vi "Billard2020.vi"() -> ()   [LabVIEW 2019]
uses:
  <vilib>/picture/picture.llb/imagedata.ctl
panel:
  in  "line":string
  in  "ball touch":u32(colorbox)
  in  "band touch":u32(colorbox)
  in  "Script":string
  out "ML":string
  out "return code":i32
  in  "Blue BG":T1={"Rmin"=39, "Rmax"=62, "Gmin"=91, "Gmax"=116, "Bmin"=202, "Bmax"=255}
  in  "White Ball":T1={"Rmin"=100, "Rmax"=255, "Gmin"=100, "Gmax"=255, "Bmin"=100, "Bmax"=255}
  in  "Yellow Ball":T1={"Rmin"=140, "Rmax"=255, "Gmin"=140, "Gmax"=255, "Bmin"=0, "Bmax"=175}
  in  "Red Ball":T1={"Rmin"=160, "Rmax"=255, "Gmin"=0, "Gmax"=160, "Bmin"=0, "Bmax"=160}
  in  "Dark Blue frame":T2={"Rmin"=0, "Gmin"=0, "Bmin"=121, "Rmax"=14, "Gmax"=42, "Bmax"=126}
  out "Bords du billard":T3
  out "filenames":string[](array[string])
  in  "path":path
  out "error out":errorcluster
  out "Ball coordinates":string
  out "standard error":string
  out "standard output":string
  out "appended array":u32[](array[numeric])
  out "H":i16
  out "W":i16
  out "2D Picture":picture
  out "image data":T4
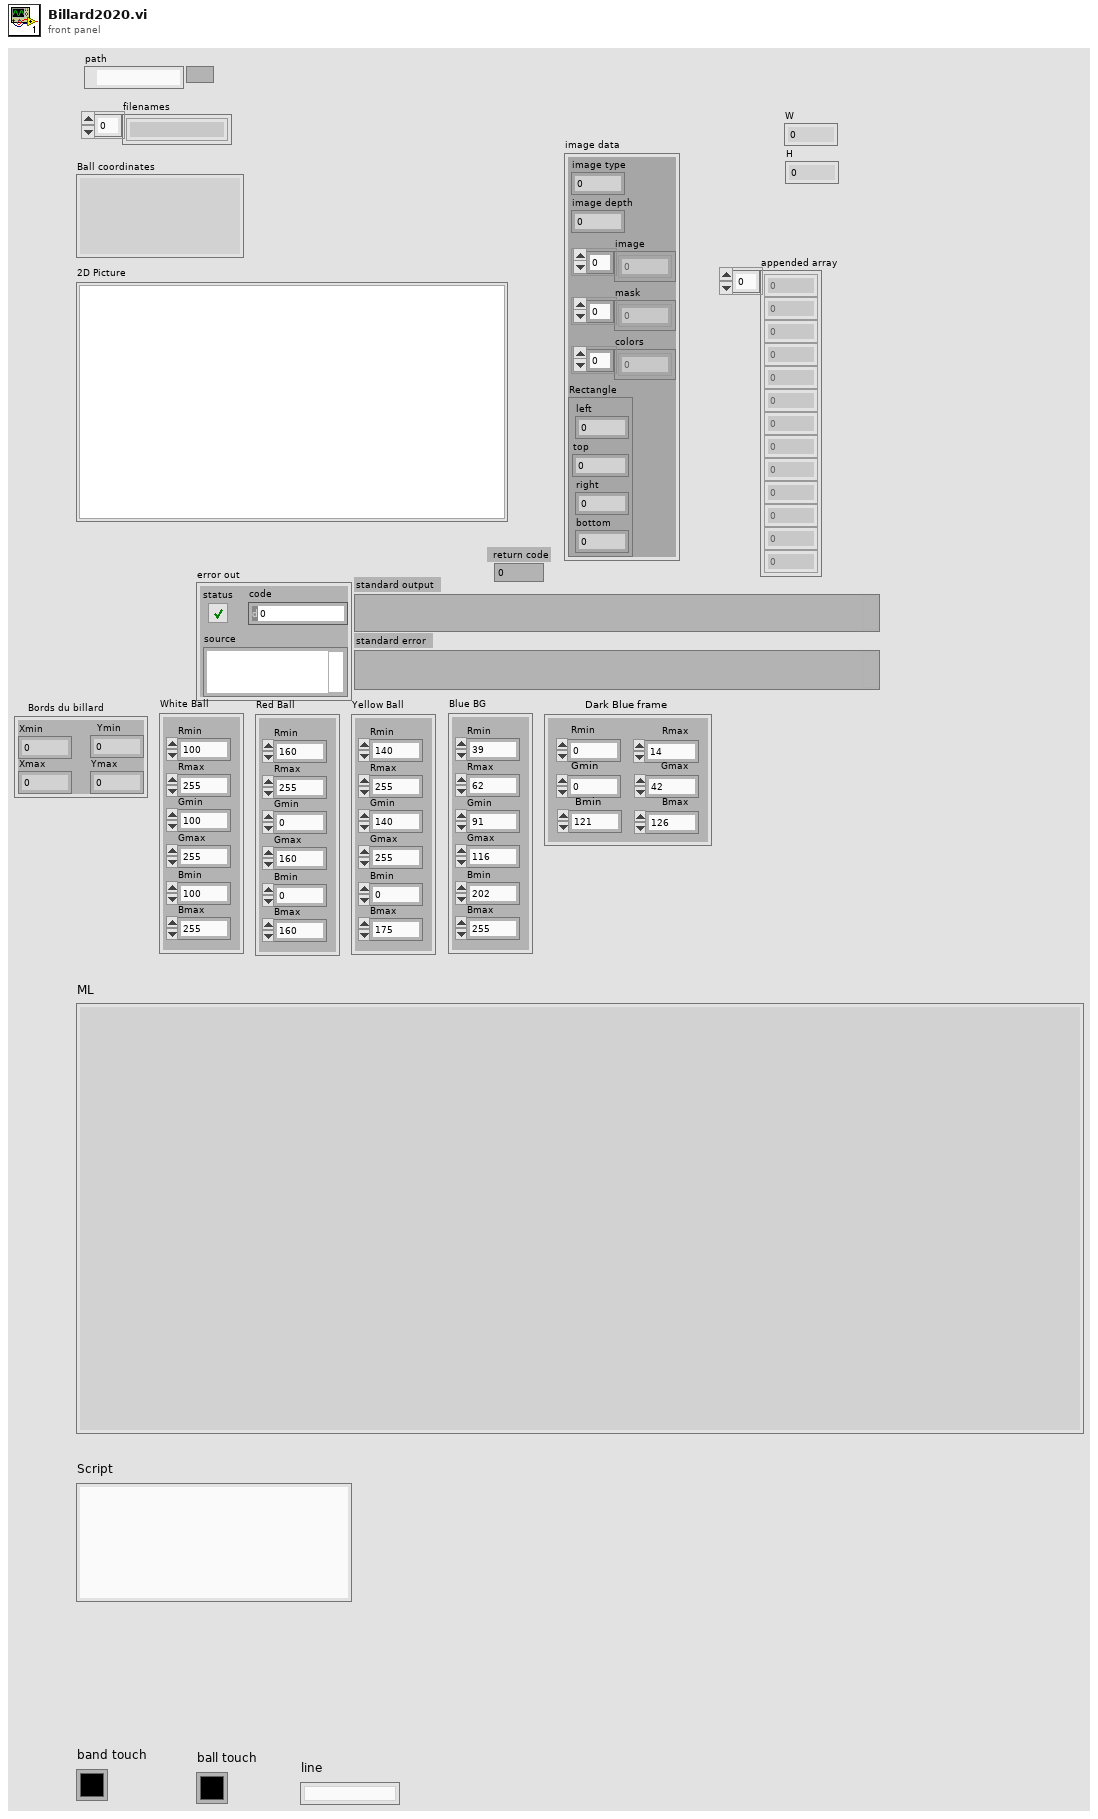
[diagram p1: front panel]
types:
  T1 = cluster{"Rmin":i32, "Rmax":i32, "Gmin":i32, "Gmax":i32, "Bmin":i32, "Bmax":i32}
  T2 = cluster{"Rmin":u32, "Gmin":u32, "Bmin":u32, "Rmax":u32, "Gmax":u32, "Bmax":u32}
  T3 = cluster{"Xmin":i32, "Ymin":i32, "Xmax":i32, "Ymax":i32}
  T4 = typedef "imagedata.ctl" = cluster{"image type":i32, "image depth":i32, "image":u8[], "mask":u8[], "colors":u32[], "Rectangle":cluster{"left":i16, "top":i16, "right":i16, "bottom":i16}}
  T5 = enum16{"big-endian, network order", "native, host order", "little-endian"}
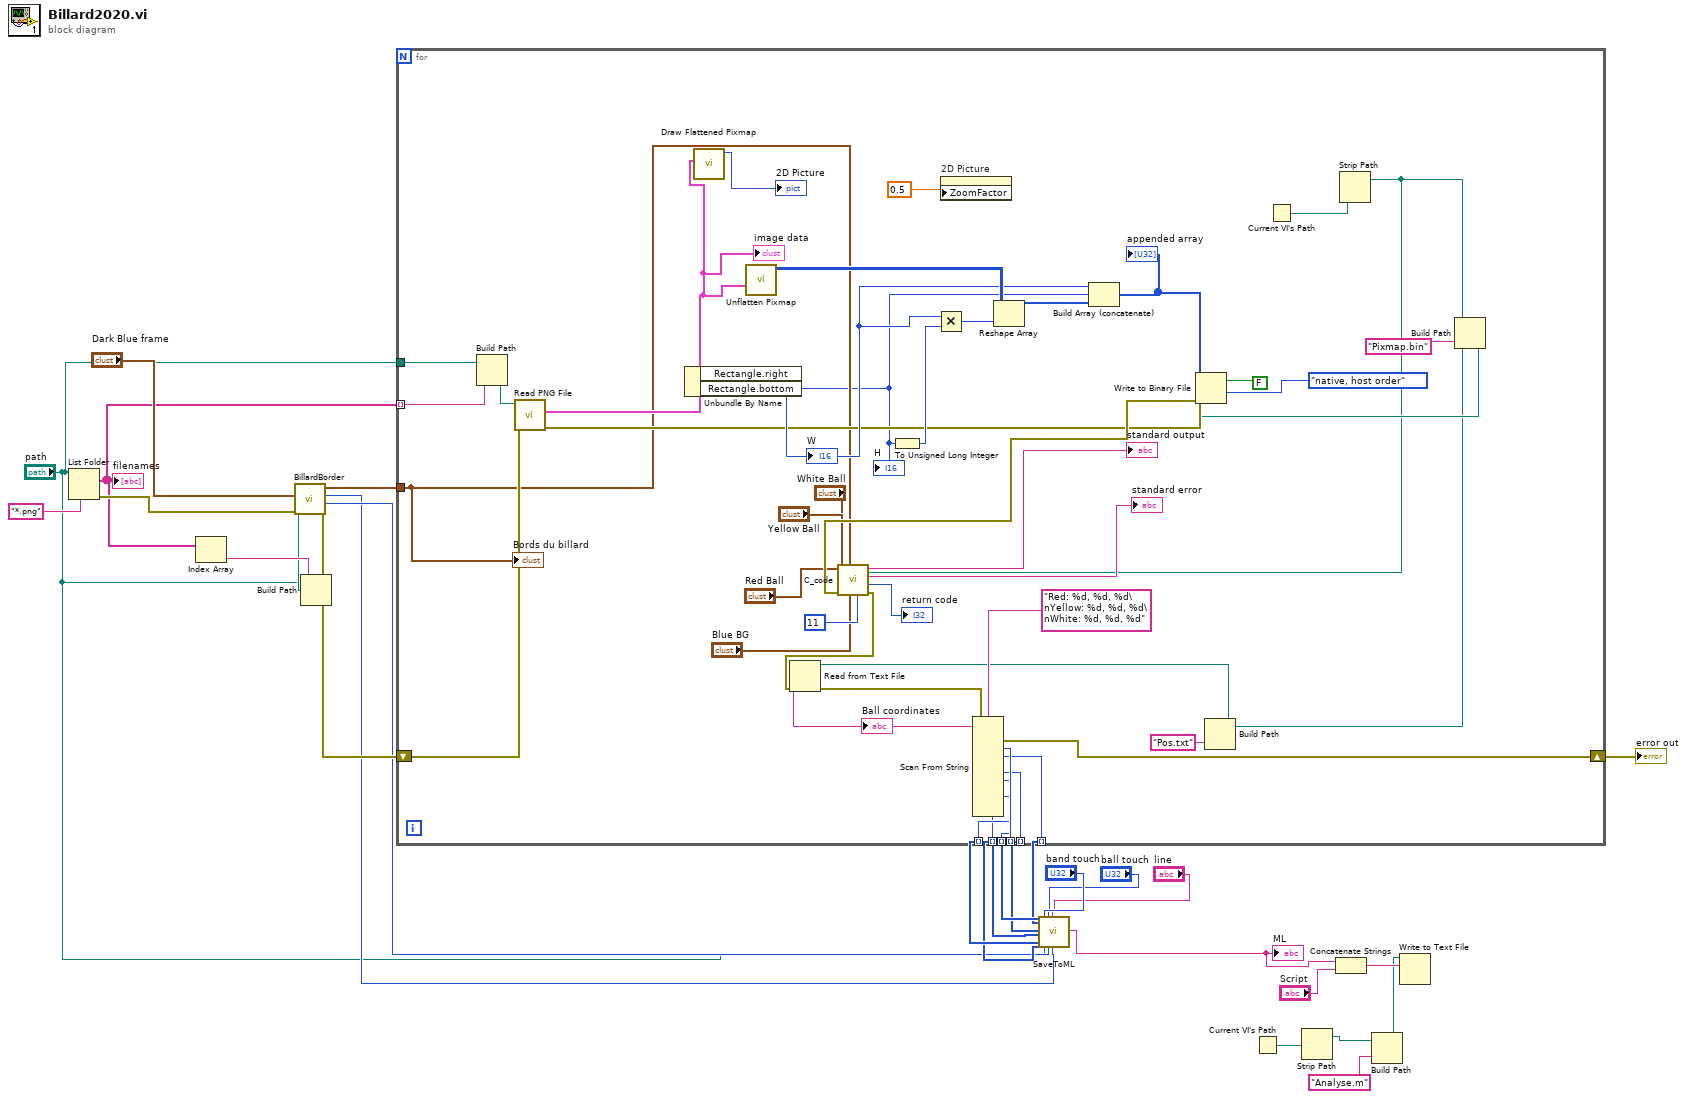
[diagram p0: block diagram]
diagram:
  n1 = List Folder(path="path", pattern="*.png") -> (filenames=w21:string[], error out=w26:errorcluster)  [unwired: 2 in, 2 out]
  "filenames" <- w21
  n2 = Index Array(array=w21) -> (element=w23:string)  [unwired: 1 in]
  n3 = Build Path(base path="path", name or relative path=w23) -> (appended path=w22:path)
  n4 = call "BillardBorder.vi"("error in (no error)"=w26, "Dark Blue frame"="Dark Blue frame", "path to PNG file"=w22) -> ("error out"=w27:errorcluster, "H"=w7:i16, "W"=w6:i16, "Bords du billard"=w24:T3)  [unwired: 5 in]
  n5 = for {
    tunnel: w24 -> [w37]
    tunnel: "path" -> [w40]
    tunnel: w21 -> [w38] mode=indexing
    shift-right: [w36] -> w14
    shift-left: w27 -> [w48]
    tunnel: [w34] -> w13 mode=indexing
    tunnel: [w33] -> w12 mode=indexing
    tunnel: [w32] -> w11 mode=indexing
    tunnel: [w31] -> w10 mode=indexing
    tunnel: [w30] -> w9 mode=indexing
    tunnel: [w29] -> w8 mode=indexing
    n6 = Build Path(base path=w40, name or relative path=w38) -> (appended path=w39:path)
    n7 = call <vilib>:"Read PNG File.vi"("error in (no error)"=w48, "path to PNG file"=w39) -> ("error out"=w55:errorcluster, "image data"=w72:T4)  [unwired: 7 in, 1 out]
    "image data" <- w72
    n8 = Unbundle By Name(w72) -> ("Rectangle.right"=w67:i16, "Rectangle.bottom"=w35:i16)
    "W" <- w67
    "H" <- w35
    n9 = call <vilib>:"Draw Flattened Pixmap.vi"("image data"=w72) -> ("new picture"=→"2D Picture":picture)  [unwired: 8 in]
    n10 = call <vilib>:"Unflatten Pixmap.vi"("image data"=w72) -> ("24-bit pixmap"=w69:u32[][])  [unwired: 4 in, 6 out]
    n11 = To Unsigned Long Integer(number=w35) -> (unsigned 32bit integer=w65:u32)
    n12 = Multiply(x=w67, y=w65) -> (x*y=w66:u32)
    n13 = property on="2D Picture" class="Pict"("ZoomFactor"=sgl 0.5 ("Zoom Factor")) -> ()  [unwired: 2 in, 2 out]
    n14 = Reshape Array(w69, w66) -> (w68:u32[])
    n15 = Build Array (concatenate)(w67, w35, w68) -> (w64:u32[])
    "appended array" <- w64
    n16 = Current VI's Path() -> (path=w53:path)
    n17 = Strip Path(path=w53) -> (stripped path=w47:path)  [unwired: 1 out]
    n18 = Build Path(base path=w47, name or relative path="Pos.txt") -> (appended path=w50:path)
    n19 = Build Path(base path=w47, name or relative path="Pixmap.bin") -> (appended path=w51:path)
    n20 = Write to Binary File(file (use dialog)=w51, data=w64, error in=w55, 5:FALSE ("prepend array or string size? (T)"), 9:T5."native, host order" ("byte order (0:big-endian, network order)")) -> (error out=w59:errorcluster)  [unwired: 1 in, 2 out]
    n21 = call "C_code.vi"("Ball Diameter"=11, "working directory"=w47, "Blue BG"="Blue BG", "Frame borders"=w37, "error in (no error)"=w59, "White Ball"="White Ball", "Yellow Ball"="Yellow Ball", "Red Ball"="Red Ball") -> ("error out"=w58:errorcluster, "return code"=→"return code":i32, "standard error"=→"standard error":string, "standard output"=→"standard output":string)
    n22 = Read from Text File(file (use dialog)=w50, error in=w58) -> (text=w57:string, error out=w54:errorcluster)  [unwired: 2 in, 2 out]
    "Ball coordinates" <- w57
    n23 = Scan From String(format string="Red: %d, %d, %d\nYellow: %d, %d, %d\nWhite: %d, %d, %d", input string=w57, error in=w54) -> (error out=w36:errorcluster, output 1=w34:i32, output 2=w33:i32, output 4=w32:i32, output 5=w31:i32, output 7=w30:i32, output 8=w29:i32)  [unwired: 13 in, 2 out]
    "Bords du billard" <- w37
  }
  "error out" <- w14
  n24 = call "SaveToML.vi"("X1"=w13, "Y1"=w12, "X2"=w11, "Y2"=w10, "X3"=w9, "Y3"=w8, "band touch"="band touch", "path"="path", "ball touch"="ball touch", "H"=w7, "line"="line", "W"=w6) -> ("ML"=w2:string)  [unwired: 15 in]
  "ML" <- w2
  n25 = Current VI's Path() -> (path=w16:path)
  n26 = Strip Path(path=w16) -> (stripped path=w15:path)  [unwired: 1 out]
  n27 = Concatenate Strings(w2, "Script") -> (w19:string)
  n28 = Build Path(base path=w15, name or relative path="Analyse.m") -> (appended path=w18:path)
  n29 = Write to Text File(file (use dialog)=w18, text=w19) -> ()  [unwired: 2 in, 3 out]
